vi "fgv_stream_w_end-pt.vi"(7 "cmd":enum16{"ini", "write", "close"}(ring), 8 "error in":errorcluster, 11 "rgb_arr":u8[](array[numeric])) -> (0 "error out":errorcluster)   [LabVIEW 2019]
uses:
  <vilib>/ErrorRing/Error Ring.xnode
  <resource>/objmgr/ni.dex.rc
panel:
  out "Write Backlog":i32
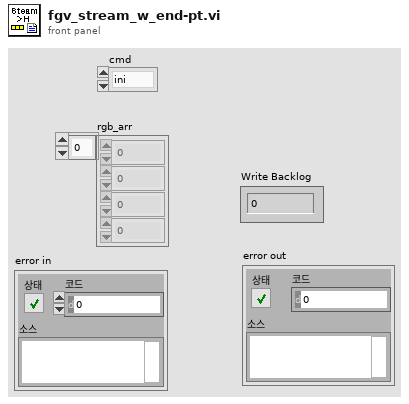
[diagram p1: front panel]
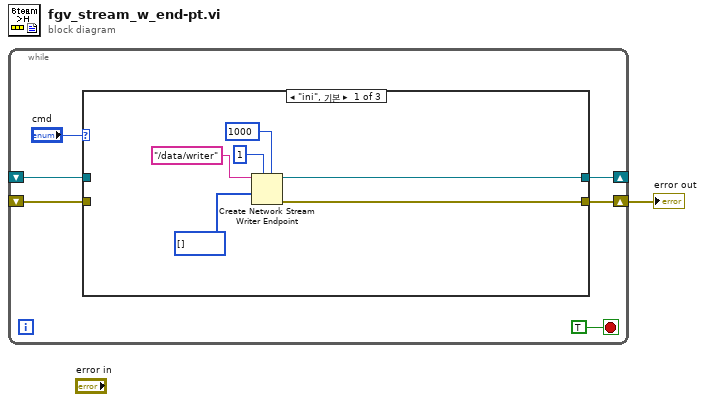
[diagram p0: block diagram]
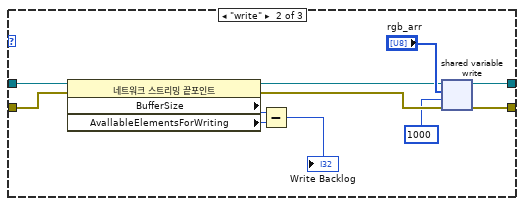
[diagram p2: hidden frame]
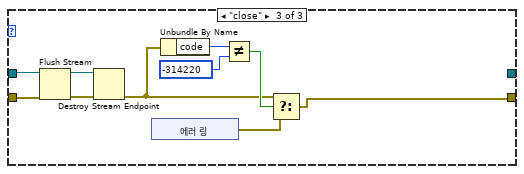
[diagram p3: hidden frame]
diagram:
  n1 = while {
    shift-right: [w4] -> _
    shift-left: _ -> [w5]
    shift-right: [w2] -> w1
    shift-left: _ -> [w3]
    stop <- TRUE stop-if-true
    n2 = case shown="\"ini\", 기본" "cmd" {
      tunnel: w5 -> [_ w17 w26]
      tunnel: [w11 w14 _] -> w4
      tunnel: w3 -> [_ w16 w27]
      tunnel: [w10 w15 w25] -> w2
      frame "ini", Default {
        n3 = Create Network Stream Writer Endpoint(5:1000 ("타임아웃(ms) (-1)"), 7:1 ("writer buffer size"), 9:u8[] [] ("imgarr"), 11:"/data/writer" ("reader url")) -> (0:w10:errorcluster, 3:w11:refnum<k21>)  [unwired: 3 in]
      }
      frame "write" {
        n4 = property class="네트워크 스트리밍 끝포인트"(reference=w17, error in=w16) -> (reference out=w22:refnum<k21>, error out=w23:errorcluster, "BufferSize"=w20:i32, "AvallableElementsForWriting"=w19:i32)
        n5 = Subtract(x=w20, y=w19) -> (x-y=→"Write Backlog":i32)
        n6 = shared-variable-write(w22, w23, "rgb_arr", 1000 ("timeout ms")) -> (w14:refnum<k21>, w15:errorcluster)  [unwired: 1 out]
      }
      frame "close" {
        n7 = Flush Stream(8:w27, 11:w26) -> (0:w33:errorcluster, 3:w34:refnum<k21>)  [unwired: 2 in, 1 out]
        n8 = Destroy Stream Endpoint(8:w33, 11:w34) -> (0:w28:errorcluster)
        n9 = xnode "에러 링"() -> ("에러 출력"=w29:errorcluster)
        n10 = Unbundle By Name(w28) -> ("code"=w32:i32)
        n11 = Not Equal?(x=w32, y=-314220) -> (x != y?=w30:bool)
        n12 = Select(t=w28, s=w30, f=w29) -> (s? t:f=w25:errorcluster)
      }
    }
  }
  "error out" <- w1
